vi "wheel mode.vi"() -> ()   [LabVIEW 2016]
uses:
  <instrlib>/Dynamixel Motor/Public/Motor Operation/Low Level/Baud Setting.ctl
  <vilib>/myRIO/Instrument Drivers/Onboard IO/DIO/typedefs/DIO Reference.ctl
  <vilib>/myRIO/Common/Instrument Driver Framework/Utilities/typedefs/myRIO Generic Hardware Reference.ctl
  <vilib>/myRIO/Common/Instrument Driver Framework/Utilities/typedefs/Hardware Version Enum.ctl
  <vilib>/myRIO/Common/Instrument Driver Framework/Utilities/typedefs/myRIO v1.0 Reference.ctl
  <vilib>/myRIO/Common/Instrument Driver Framework/Utilities/typedefs/Generic FPGA Reference.ctl
  <vilib>/myRIO/Common/Instrument Driver Framework/myRIO v1.0/DIO/typedefs/DIO Channels List.ctl
  <vilib>/myRIO/Common/Instrument Driver Framework/myRIO v1.0/DIO/typedefs/DIO Channels Enum.ctl
  <vilib>/userdefined/High Color/nirio_resource_hc.ctl
  <vilib>/myRIO/Common/Instrument Driver Framework/Utilities/vis/Is FPGA Ref Available.vi
  <vilib>/myRIO/Common/Instrument Driver Framework/myRIO v1.0/DIO/vis/myRIO v1.1 Open DIO.vi
  <vilib>/myRIO/Instrument Drivers/Onboard IO/DIO/vis/Write.vi
  <vilib>/myRIO/Common/Instrument Driver Framework/Utilities/vis/Validate Channels.vi
  <vilib>/myRIO/Common/Instrument Driver Framework/myRIO v1.0/DIO/vis/myRIO v1.0 Reserve DIO.vi
  <vilib>/myRIO/Common/Instrument Driver Framework/myRIO v1.0/UART/vis/myRIO v1.0 Close UART.vi
  <vilib>/myRIO/Common/Instrument Driver Framework/myRIO v1.0/Resource Manager/vis/myRIO v1.0 Reserve Channel List.vi
  <vilib>/myRIO/Common/Instrument Driver Framework/myRIO v1.0/DIO/vis/myRIO v1.0 Build MUX Configuration DIO.vi
  <vilib>/myRIO/Common/Instrument Driver Framework/myRIO v1.0/Resource Manager/vis/myRIO v1.0 Reserve Channel.vi
  <vilib>/myRIO/Common/Instrument Driver Framework/myRIO v1.0/Resource Manager/vis/myRIO v1.0 Unreserve Channel.vi
  <vilib>/myRIO/Common/Instrument Driver Framework/myRIO v1.0/Resource Manager/vis/myRIO v1.0 Create Configuration List.vi
  <vilib>/myRIO/Common/Instrument Driver Framework/myRIO v1.0/Resource Manager/vis/myRIO v1.0 Build Mutex Name.vi
  <vilib>/Utility/VariantDataType/GetNumericInfo.vi
  <vilib>/Utility/error.llb/Error Cluster From Error Code.vi
  <vilib>/myRIO/Common/Instrument Driver Framework/myRIO v1.0/myRIO v1.1 Open.vi
  <vilib>/myRIO/Common/Instrument Driver Framework/Utilities/vis/IO Manager.vi
  <vilib>/myRIO/Common/Instrument Driver Framework/Utilities/vis/Configuration Manager.vi
  <vilib>/myRIO/Common/Instrument Driver Framework/myRIO v1.0/Resource Manager/vis/myRIO v1.0 Configure IO.vi
  <vilib>/myRIO/Common/Instrument Driver Framework/myRIO v1.0/myRIO v1.0 Close.vi
  <vilib>/myRIO/Common/Instrument Driver Framework/myRIO v1.0/DIO/vis/myRIO v1.0 Write DIO.vi
  <vilib>/myRIO/Common/Instrument Driver Framework/Utilities/vis/FPGA Ref Manager.vi
  <vilib>/myRIO/Common/Instrument Driver Framework/myRIO v1.0/myRIO v1.0 Reset FPGA.vi
  <vilib>/myRIO/Common/Instrument Driver Framework/myRIO v1.0/IRQ/vis/myRIO v1.0 IRQ Info FGV.vi
  <vilib>/myRIO/Common/Instrument Driver Framework/myRIO v1.0/IRQ/vis/myRIO v1.0 Timer IRQ Info FGV.vi
  <vilib>/myRIO/Common/Instrument Driver Framework/myRIO v1.0/IRQ/vis/myRIO v1.0 ISR Agent.vi
  <vilib>/myRIO/Express VI/Onboard Devices/LED/LED Express VI.xnode
  <vilib>/myRIO/Instrument Drivers/Onboard IO/DIO/vis/myRIO DIO Open.xnode
  <instrlib>/Dynamixel Motor/Dynamixel Motor.lvlib
  <vilib>/myRIO/Instrument Drivers/Onboard IO/DIO/DIO.lvlib
  <vilib>/myRIO/Instrument Drivers/Utilities/Utilities.lvlib
panel:
  in  "LED0":bool
  in  "Goal Speed (RPM)":dbl
  out "Load/torque %":sgl
  in  "Motor ID (0)":u8=5
  in  "정지":bool
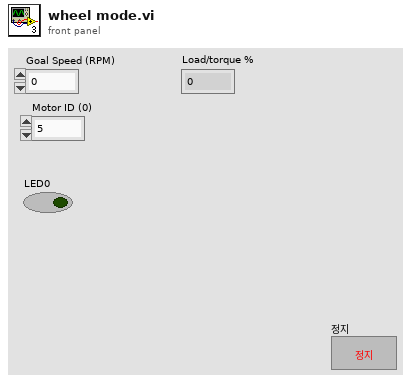
[diagram p1: front panel]
types:
  T1 = typedef "Dynamixel Motor.lvlib/Baud Setting.ctl" = u8
  T2 = typedef "DIO.lvlib/DIO Reference.ctl" = cluster{"myRIO Reference":T3, "DIO Channels List":T7}
  T3 = typedef "myRIO Generic Hardware Reference.ctl" = cluster{"myRIO Model":T4, "myRIO Hardware Reference":T5}
  T4 = typedef "Hardware Version Enum.ctl" = enum16{"Unknown", "myRIO-1900", "myRIO-1950", "roboRIO", "NI ELVIS RIO CM"}
  T5 = typedef "myRIO v1.0 Reference.ctl" = cluster{"Generic FPGA Reference":T6, "Allow multiple opens":bool}
  T6 = typedef "Generic FPGA Reference.ctl" = refnum<k20>
  T7 = typedef "DIO Channels List.ctl" = T8[]
  T8 = typedef "DIO Channels Enum.ctl" = enum16{"Not Connected", "C/DIO0", "C/DIO1", "C/DIO2", "C/DIO3", "C/DIO4", "C/DIO5", "C/DIO6", "C/DIO7", "A/DIO0", "A/DIO1", "A/DIO2", "A/DIO3", "A/DIO4", "A/DIO5", "A/DIO6", "A/DIO7", "A/DIO8", "A/DIO9", "A/DIO10", "A/DIO11", "A/DIO12", "A/DIO13", "A/DIO14", "A/DIO15", "B/DIO0", "B/DIO1", "B/DIO2", "B/DIO3", "B/DIO4", "B/DIO5", "B/DIO6", "B/DIO7", "B/DIO8", "B/DIO9", "B/DIO10", "B/DIO11", "B/DIO12", "B/DIO13", "B/DIO14", "B/DIO15", "LED0", "LED1", "LED2", "LED3", "Button0", "DIO/DIO0", "DIO/DIO1", "DIO/DIO2", "DIO/DIO3", "DIO/DIO4", "DIO/DIO5", "DIO/DIO6", "DIO/DIO7", "DIO/DIO8", "DIO/DIO9", "SPI/CS0", "SPI/CS1", "SPI/CS2", "SPI/CS3", "LED RADIO (Green)", "LED RADIO (Red)", "LED COMM (Green)", "LED COMM (Red)", "LED MODE (Green)", "LED MODE (Red)"}
  T9 = typedef "nirio_resource_hc.ctl" = tag
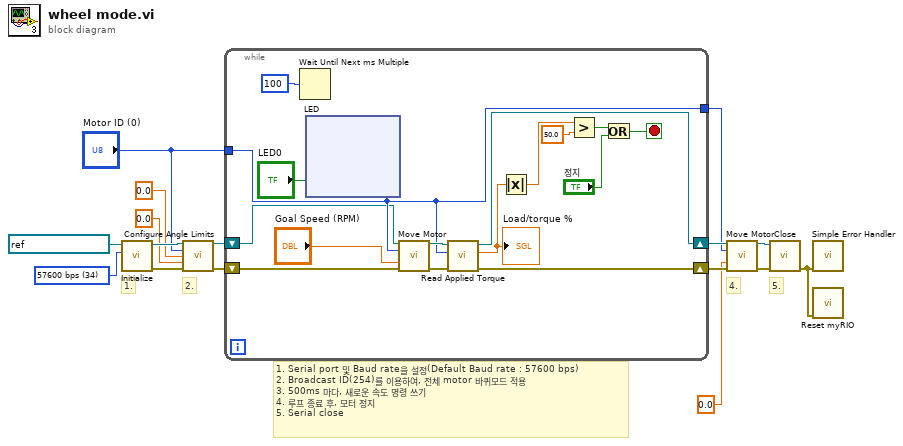
[diagram p0: block diagram]
diagram:
  w15 = T1 34 items=["1,000,000 bps"=1, "500,000 bps"=3, "400,000 bps"=4, "250,000 bps"=7, "200,000 bps"=9, "115200 bps"=16, "57600 bps"=34, "19200 bps"=103, "9600 bps"=207] ("Baud rate (57600 bps)")
  # "5."
  # "1. Serial port 및 Baud rate을 설정(Default Baud rate : 57600 bps)\n2. Broadcast ID(254)를 이용하여, 전체 motor 바퀴모드 적용\n3. 500ms 마다, 새로운 속도 명령 쓰기\n4. 루프 종료 후, 모터 정지\n5. Serial close"
  # "2."
  # "4."
  # "1."
  n1 = call <instrlib>:"Initialize.vi"("Baud rate (57600 bps)"=w15, "VISA resource name"=refnum<visa-resource-name> "ASRL3::INSTR") -> ("error out"=w16:errorcluster, "VISA resource name out"=w8:refnum<visa-resource-name>)  [unwired: 8 in]
  n2 = call <instrlib>:"Configure Angle Limits.vi"("VISA resource name"=w8, "Motor ID (0)"="Motor ID (0)", "Clockwise Angle Limit (0 deg)"=0.0, "Counter-Clockwise Angle Limit (300 deg)"=0.0, "error in (no error)"=w16) -> ("VISA resource name out"=w14:refnum<visa-resource-name>, "error out"=w13:errorcluster)  [unwired: 9 in]
  n3 = while {
    shift-right: [w28] -> w11
    shift-left: w14 -> [w25]
    shift-right: [w29] -> w10
    shift-left: w13 -> [w26]
    tunnel: "Motor ID (0)" -> [w27]
    tunnel: [w27] -> w4
    stop <- w19 stop-if-true
    n4 = Wait Until Next ms Multiple(millisecond multiple=u32 100 ("ms 배수")) -> ()  [unwired: 1 out]
    n5 = xnode "LED"("LED0"="LED0") -> ()  [unwired: 1 in, 1 out]
    n6 = call <instrlib>:"Move Motor.vi"("VISA resource name"=w25, "Motor ID (0)"=w27, "Goal Speed (RPM)"="Goal Speed (RPM)", "error in (no error)"=w26) -> ("VISA resource name out"=w31:refnum<visa-resource-name>, "error out"=w30:errorcluster)  [unwired: 10 in]
    n7 = call <instrlib>:"Read Applied Torque.vi"("error in (no error)"=w30, "Motor ID (0)"=w27, "VISA resource name"=w31) -> ("error out"=w29:errorcluster, "Load/torque %"=w18:sgl, "VISA resource name out"=w28:refnum<visa-resource-name>)  [unwired: 6 in]
    "Load/torque %" <- w18
    n8 = Absolute Value(x=w18) -> (abs(x)=w17:sgl)
    n9 = Greater?(x=w17, y=sgl 50.0) -> (0:w21:bool)
    n10 = Or(x=w21, y="정지") -> (x .or. y?=w19:bool)
  }
  n11 = call <instrlib>:"Move Motor.vi"("VISA resource name"=w11, "Motor ID (0)"=w4, "Goal Speed (RPM)"=0.0 ("Goal Position (180 deg)"), "error in (no error)"=w10) -> ("VISA resource name out"=w9:refnum<visa-resource-name>, "error out"=w12:errorcluster)  [unwired: 10 in]
  n12 = call <instrlib>:"Close.vi"("error in (no error)"=w12, "VISA resource name"=w9) -> ("error out"=w1:errorcluster)  [unwired: 9 in]
  n13 = call <vilib>:"Simple Error Handler.vi"("error in (no error)"=w1) -> ()  [unwired: 4 in, 5 out]
  n14 = call <vilib>:"Reset myRIO.vi"("error in (no error)"=w1) -> ()  [unwired: 10 in, 1 out]
